vi "Get Temp Ramp Rate--Method.vi"(8 "error in (no error)":errorcluster, 10 "Temp Ramp Data":T1, 11 "Simulated Thermal Process Controller in":refnum<class "Simulated Thermal Process Controller.lvclass">) -> (0 "error out":errorcluster, 2 "Temp Ramp Rate":dbl, 3 "Simulated Thermal Process Controller out":refnum<class "Simulated Thermal Process Controller.lvclass">)   [LabVIEW 2024, in "Simulated Thermal Process Controller.lvclass"]
uses:
  Simulated Thermal Process Controller.lvclass
  Process Controller/Controls/Temp Ramp Rate Data--Cluster.ctl
  Process Controller/Controls/Temperature Units--Enum.ctl
  Process Controller/Controls/Rate Units--Enum.ctl
  Simulated Thermal Process Controller.lvclass/Simulated Thermal Process Controller.ctl
  Process Controller/_Thermal Process Controller.lvclass
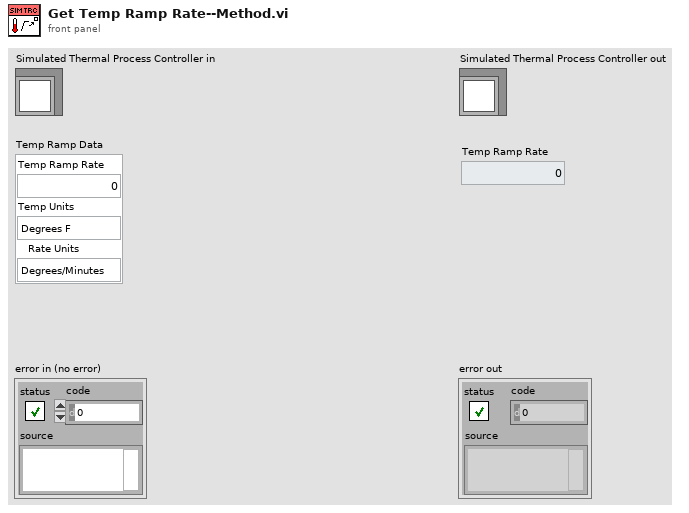
[diagram p1: front panel]
types:
  T1 = typedef "_Thermal Process Controller.lvclass/Temp Ramp Rate Data--Cluster.ctl" = cluster{"Temp Ramp Rate":dbl, "Temp Units":T2, "Rate Units":T3}
  T2 = typedef "_Thermal Process Controller.lvclass/Temperature Units--Enum.ctl" = enum16{"Degrees F", "Degrees C", "Degrees K"}
  T3 = typedef "_Thermal Process Controller.lvclass/Rate Units--Enum.ctl" = enum16{"Degrees/Minutes", "Degrees/Hours"}
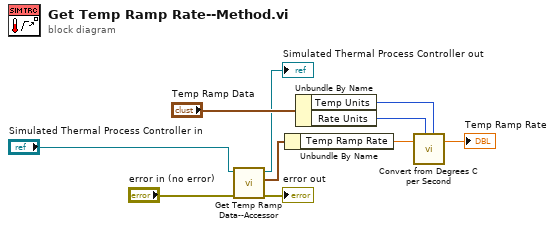
[diagram p0: block diagram]
diagram:
  n1 = call "Get Temp Ramp Data--Accessor.vi"("error in (no error)"="error in (no error)", "Simulated Thermal Process Controller in"="Simulated Thermal Process Controller in") -> ("error out"=→"error out":errorcluster, "Temp Ramp Data"=w7:T1, "Simulated Thermal Process Controller out"=→"Simulated Thermal Process Controller out":refnum<class "Simulated Thermal Process Controller.lvclass">)  [unwired: 7 in]
  n2 = Unbundle By Name(w7) -> ("Temp Ramp Rate"=w2:dbl)
  n3 = Unbundle By Name("Temp Ramp Data") -> ("Temp Units"=w3:T2, "Rate Units"=w4:T3)
  n4 = call "Convert from Degrees C per Second.vi"("Rate In"=w2, "Rate Units"=w4, "Temp Units"=w3) -> ("Rate Out"=→"Temp Ramp Rate":dbl)  [unwired: 4 in]
